vi "Initialize.vi"(8 "error in (no error)":errorcluster, 11 "Flip Mirror Containter in":refnum<class "Flip Mirror Containter.lvclass">) -> (0 "error out":errorcluster, 3 "Flip Mirror Containter out":refnum<class "Flip Mirror Containter.lvclass">)   [LabVIEW 2016, in "Flip Mirror Containter.lvclass"]
uses:
  Flip Mirror Containter.lvclass
  ExtFlatMir.lvclass
  SolarMir.lvclass
  ThArMir.lvclass
  Flip Mirror Containter.lvclass/Flip Mirror Containter.ctl
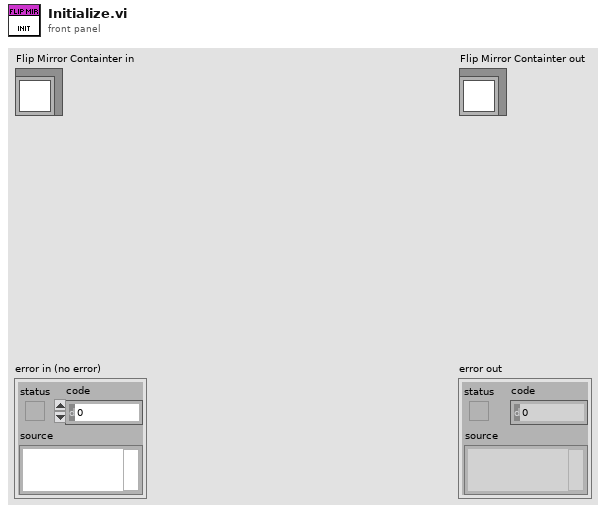
[diagram p1: front panel]
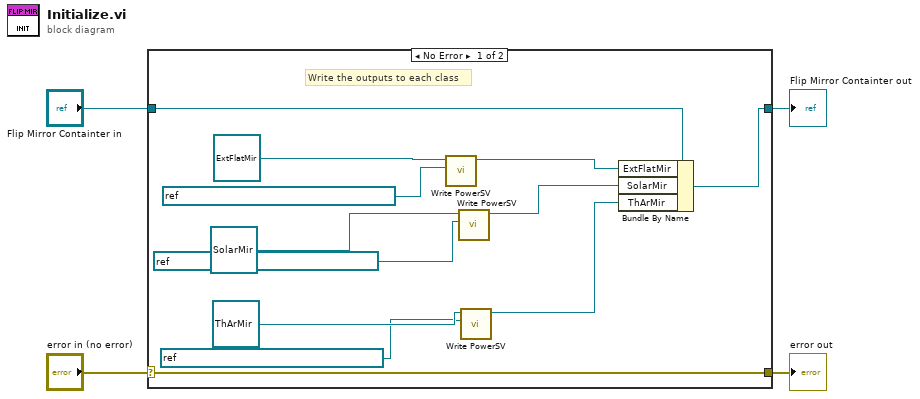
[diagram p0: block diagram]
diagram:
  n1 = case shown="No Error" "error in (no error)" {
    selector: "error in (no error)" -> [w16 w18]
    tunnel: [w16 w18] -> w3
    tunnel: [w12 w17] -> w1
    tunnel: "Flip Mirror Containter in" -> [w13 w17]
    frame No Error {
      # "Write the outputs to each class"
      n2 = call-dynamic "Write PowerSV.vi"("PowerSV"=refnum<k21> "ni.var.io://bem-rt/Mod2/ExtFlatMirOut", "FlipMir in"=refnum<class "ExtFlatMir.lvclass"> refnum ("ExtFlatMir.lvclass")) -> ("FlipMir out"=w11:refnum<class "ExtFlatMir.lvclass">)  [unwired: 8 in, 1 out]
      n3 = call-dynamic "Write PowerSV.vi"("PowerSV"=refnum<k21> "ni.var.io://bem-rt/Mod2/SolarMirOut", "FlipMir in"=refnum<class "SolarMir.lvclass"> refnum ("SolarMir.lvclass")) -> ("FlipMir out"=w6:refnum<class "SolarMir.lvclass">)  [unwired: 8 in, 1 out]
      n4 = call-dynamic "Write PowerSV.vi"("PowerSV"=refnum<k21> "ni.var.io://bem-rt/Mod2/TharMirOut", "FlipMir in"=refnum<class "ThArMir.lvclass"> refnum ("ThArMir.lvclass")) -> ("FlipMir out"=w7:refnum<class "ThArMir.lvclass">)  [unwired: 8 in, 1 out]
      n5 = Bundle By Name(cluster=w13, "ExtFlatMir"=w11, "SolarMir"=w6, "ThArMir"=w7) -> (w12:refnum<class "Flip Mirror Containter.lvclass">)
    }
    frame Error {
    }
  }
  "error out" <- w3
  "Flip Mirror Containter out" <- w1
